vi "Shift Fwd.vi"(10 "iterator":refnum<data-value>, 11 "Node in":refnum<class "Node.lvclass">) -> (3 "Node out":refnum<class "Node.lvclass">)   [LabVIEW 2023, in "d20.lvlib" / "Node.lvclass"]
uses:
  Node.lvclass
  INode/INode.lvclass
  Node.lvclass/Node.ctl
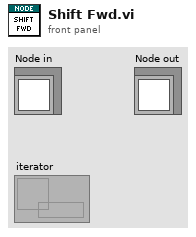
[diagram p1: front panel]
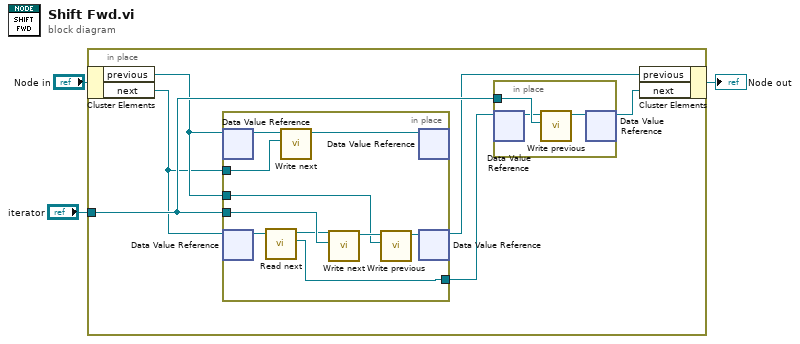
[diagram p0: block diagram]
diagram:
  n1 = in-place {
    in-place-border: "iterator" -> [w9]
    n2 = in-place-cluster #1("Node in") -> ("previous"=w7:refnum<data-value>, "next"=w5:refnum<data-value>)
    n3 = in-place {
      in-place-border: w7 -> [w16]
      in-place-border: [w20] -> w8
      in-place-border: w5 -> [w22]
      in-place-border: w9 -> [w19]
      n4 = in-place-dvr #2(w7) -> (w13:refnum<class "INode.lvclass">)  [unwired: 1 out]
      n5 = in-place-dvr #3(w5) -> (w14:refnum<class "INode.lvclass">)  [unwired: 1 out]
      n6 = call-dynamic "Read next.vi"("Node in"=w14) -> ("next"=w20:refnum<data-value>, "Node out"=w18:refnum<class "INode.lvclass">)  [unwired: 9 in]
      n7 = call-dynamic "Write next.vi"("next"=w22, "Node in"=w13) -> ("Node out"=w21:refnum<class "INode.lvclass">)  [unwired: 9 in]
      n8 = call-dynamic "Write next.vi"("next"=w19, "Node in"=w18) -> ("Node out"=w17:refnum<class "INode.lvclass">)  [unwired: 9 in]
      n9 = call-dynamic "Write previous.vi"("previous"=w16, "Node in"=w17) -> ("Node out"=w15:refnum<class "INode.lvclass">)  [unwired: 9 in]
      n10 = in-place-dvr #2(w21) -> ()  [unwired: 2 out]
      n11 = in-place-dvr #3(w15) -> (w4:refnum<data-value>)  [unwired: 1 out]
    }
    n12 = in-place {
      in-place-border: w9 -> [w12]
      n13 = in-place-dvr #4(w8) -> (w11:refnum<class "INode.lvclass">)  [unwired: 1 out]
      n14 = call-dynamic "Write previous.vi"("previous"=w12, "Node in"=w11) -> ("Node out"=w10:refnum<class "INode.lvclass">)  [unwired: 9 in]
      n15 = in-place-dvr #4(w10) -> (w6:refnum<data-value>)  [unwired: 1 out]
    }
    n16 = in-place-cluster #1("previous"=w4, "next"=w6) -> (→"Node out":refnum<class "Node.lvclass">)
  }
